vi "LJM_LoadConstants.vi"   [LabVIEW 2024]
uses:
  labjackm.dll
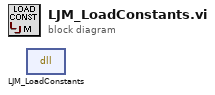
[diagram p0: block diagram]
diagram:
  n1 = dll-call lib="labjackm.dll" fn="LJM_LoadConstants"() -> ()  [unwired: 4 in, 2 out]
